vi "PI Query.vi"(0 "System no.":i32=1 min=1 step=1, 1 "Error check settings":T1(ring)=enum."Use global settings", 2 "String to send":string, 3 "Attach termination char.?":bool=TRUE, 4 "Strip spaces?":bool, 5 "error in":errorcluster, 7 "Delay before error check (ms)":u32) -> (14 "String read":string, 15 "bytes read":u16, 16 "Controller error":bool, 19 "error out":errorcluster)   [LabVIEW 2020]
doc: "This VI acquires the semaphore for the corresponding system via PI acquire semaphore.vi, sends a string w/o termination character via the selected interface, receives the answer and releases the semaphore via PI release semaphore.vi"
uses:
  Global1.vi
panel:
  # "This vi sends a string w/o termination character via the selected interface and receives the answer."
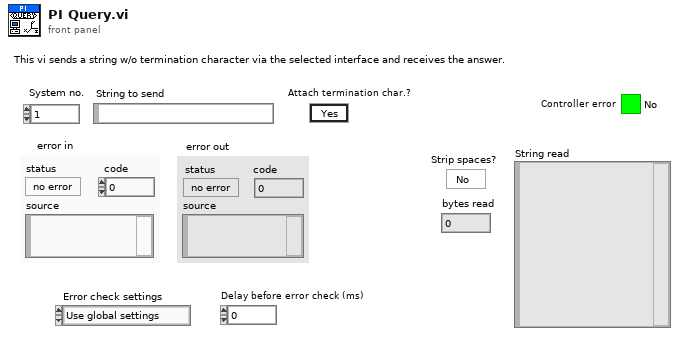
[diagram p1: front panel]
types:
  T1 = enum16{"Disable error check", "Force error check", "Use global settings"}
  T2 = typedef "Semaphore RefNum" = refnum<k1>
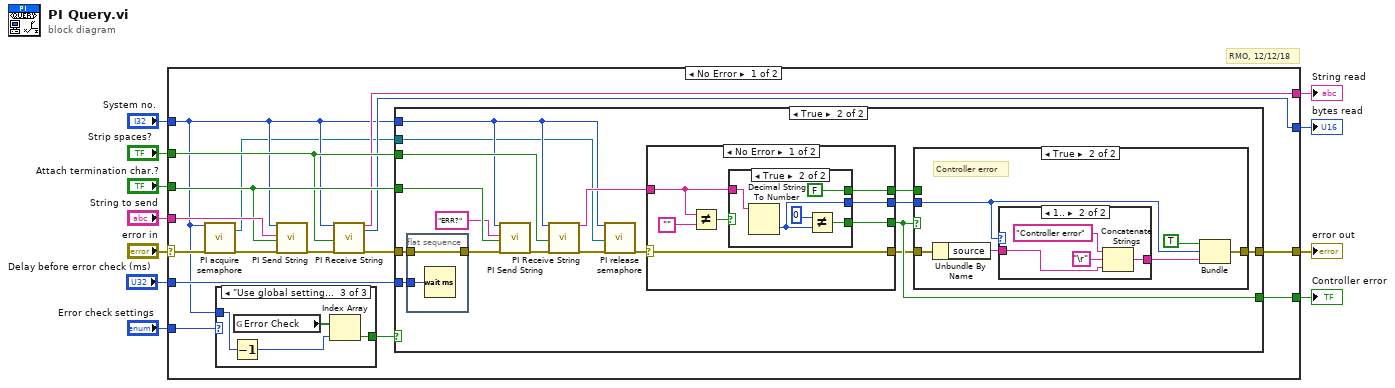
[diagram p0: block diagram]
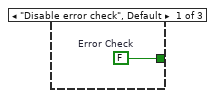
[diagram p2: hidden frame]
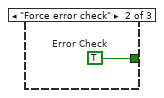
[diagram p3: hidden frame]
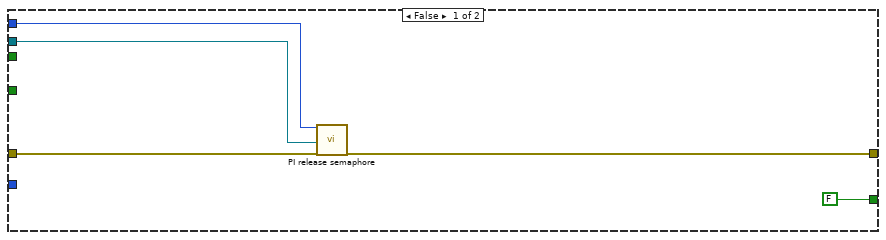
[diagram p4: hidden frame]
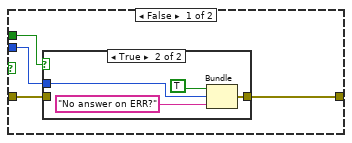
[diagram p5: hidden frame]
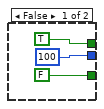
[diagram p8: hidden frame]
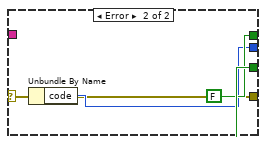
[diagram p9: hidden frame]
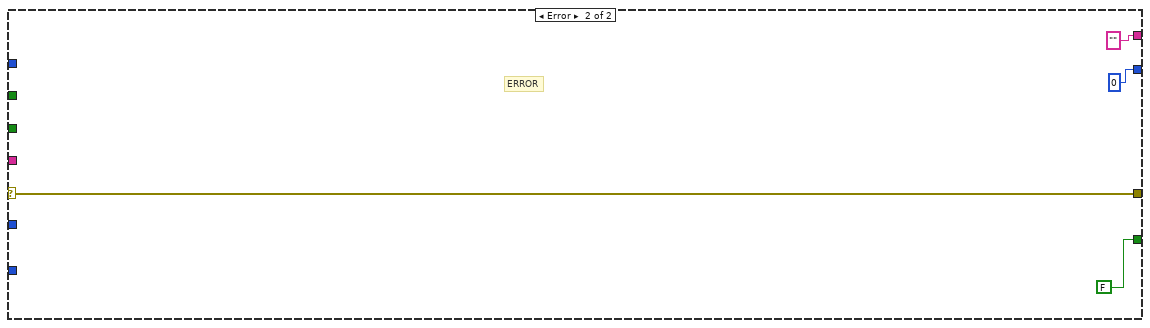
[diagram p10: hidden frame]
diagram:
  # "RMO, 12/12/18"
  n1 = case shown="No Error" "error in" {
    selector: "error in" -> [w15 w98]
    tunnel: [w27 w98] -> w3
    tunnel: "String to send" -> [w24 _]
    tunnel: "Attach termination char.?" -> [w23 _]
    tunnel: "Strip spaces?" -> [w22 _]
    tunnel: "System no." -> [w13 _]
    tunnel: [w21 "" ("String read")] -> w8
    tunnel: [w20 u16 0 ("bytes read")] -> w7
    tunnel: "Delay before error check (ms)" -> [w19 _]
    tunnel: "Error check settings" -> [w17 _]
    tunnel: [w16 FALSE] -> w2
    frame No Error {
      n2 = call "PI acquire semaphore.vi"("System no."=w13, "error in"=w15) -> ("semaphore out"=w12:T2, "error out"=w14:errorcluster)  [unwired: 16 out]
      n3 = case shown="\"Use global settings\"" w17 {
        tunnel: w13 -> [_ _ w32]
        tunnel: [w28 w29 w30] -> w18
        frame "Disable error check", Default {
          w28 = FALSE  # Error Check
        }
        frame "Force error check" {
          w29 = TRUE  # Error Check
        }
        frame "Use global settings" {
          n4 = Decrement(x=w32) -> (x-1=w31:i32)
          n5 = global read "Global1.vi" "Error Check"() -> (w33:bool[])
          n6 = Index Array(array=w33, index=w31) -> (element=w30:bool)
        }
      }
      n7 = call "PI Send String.vi"("System no."=w13, "String to send"=w24, "Attach termination char.?"=w23, "error in"=w14) -> ("error out"=w26:errorcluster)  [unwired: 15 out]
      n8 = call "PI Receive String.vi"("System no."=w13, "Strip spaces?"=w22, "error in"=w26) -> ("String read"=w21:string, "bytes read"=w20:u16, "error out"=w25:errorcluster)  [unwired: 14 out]
      n9 = case shown="True" w18 {
        tunnel: w25 -> [w38 w47]
        tunnel: [w36 w53] -> w27
        tunnel: w13 -> [w37 w43]
        tunnel: w23 -> [_ w51]
        tunnel: w22 -> [_ w50]
        tunnel: w19 -> [_ w45]
        tunnel: w12 -> [w35 w42]
        tunnel: [FALSE w41] -> w16
        frame False {
          n10 = call "PI release semaphore.vi"("System no."=w37, "semaphore"=w35, "error in"=w38) -> ("error out"=w36:errorcluster)  [unwired: 1 in, 15 out]
        }
        frame True {
          n11 = flat-sequence {
            tunnel: w47 -> [w57]
            tunnel: [w57] -> w46
            tunnel: w45 -> [w56]
            frame #0 {
              n12 = Wait (ms)(milliseconds to wait=w56) -> ()  [unwired: 1 out]
            }
          }
          n13 = call "PI Send String.vi"("System no."=w43, "String to send"="ERR?", "Attach termination char.?"=w51, "error in"=w46) -> ("error out"=w52:errorcluster)  [unwired: 15 out]
          n14 = call "PI Receive String.vi"("System no."=w43, "Strip spaces?"=w50, "error in"=w52) -> ("String read"=w48:string, "error out"=w44:errorcluster)  [unwired: 15 out]
          n15 = call "PI release semaphore.vi"("System no."=w43, "semaphore"=w42, "error in"=w44) -> ("error out"=w40:errorcluster)  [unwired: 1 in, 15 out]
          n16 = case shown="No Error" w40 {
            selector: w40 -> [w78 w93]
            tunnel: w48 -> [w82 _]
            tunnel: [w84 FALSE ("Controller Error")] -> w41
            tunnel: [w83 w94] -> w55
            tunnel: [w79 FALSE ("Controller Error")] -> w54
            tunnel: [w78 w93] -> w39
            frame No Error {
              n17 = Not Equal?(x=w82, y="") -> (x != y?=w81:bool)
              n18 = case shown="True" w81 {
                tunnel: [FALSE w92] -> w84
                tunnel: w82 -> [_ w90]
                tunnel: [100 w89] -> w83
                tunnel: [TRUE FALSE] -> w79
                frame False {
                }
                frame True {
                  n19 = Decimal String To Number(string=w90) -> (number=w89:i32)  [unwired: 3 out]
                  n20 = Not Equal?(x=0, y=w89) -> (x != y?=w92:bool)
                }
              }
            }
            frame Error {
              n21 = Unbundle By Name(w93) -> ("code"=w94:i32)
            }
          }
          n22 = case shown="True" w41 {
            tunnel: w55 -> [w58 w70]
            tunnel: [w60 w72] -> w53
            tunnel: w39 -> [w61 w68]
            tunnel: w54 -> [w59 _]
            frame False {
              n23 = case shown="True" w59 {
                tunnel: w61 -> [w62 _]
                tunnel: [w62 w63] -> w60
                tunnel: w58 -> [_ w65]
                frame False {
                }
                frame True {
                  n24 = Bundle("status"=TRUE, "code"=w65, "No answer on ERR?") -> (w63:cluster{"status":bool, "code":i32, string})  [unwired: 1 out]
                }
              }
            }
            frame True {
              # "Controller error"
              n25 = Unbundle By Name(w68) -> ("source"=w67:string)
              n26 = case shown="1.." w70 {
                tunnel: [w73 w77] -> w69
                tunnel: w67 -> [w73 w75]
                frame ..0 {
                }
                frame 1.. {
                  n27 = Concatenate Strings("Controller error", "\r" ("Substring"), w75) -> (w77:string)
                }
              }
              n28 = Bundle("status"=TRUE, "code"=w70, "source"=w69) -> (w72:errorcluster)  [unwired: 1 out]
            }
          }
        }
      }
    }
    frame Error {
      # "ERROR"
    }
  }
  "error out" <- w3
  "String read" <- w8
  "bytes read" <- w7
  "Controller error" <- w2
